vi "CRYCurve complex averaging real-time fft.vi"(7 "Initialize (F)":bool, 8 "Exponential averaging? (F=linear)":bool, 10 "Number of averages (no change)":i32, 11 "Input curve, complex":cdb[](array[numeric]) format="%.2f") -> (3 "Averaged curve":dbl[](array[numeric]) format="%.2f")   [LabVIEW 2013]
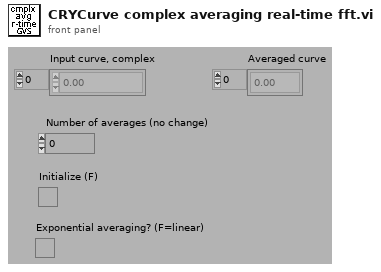
[diagram p1: front panel]
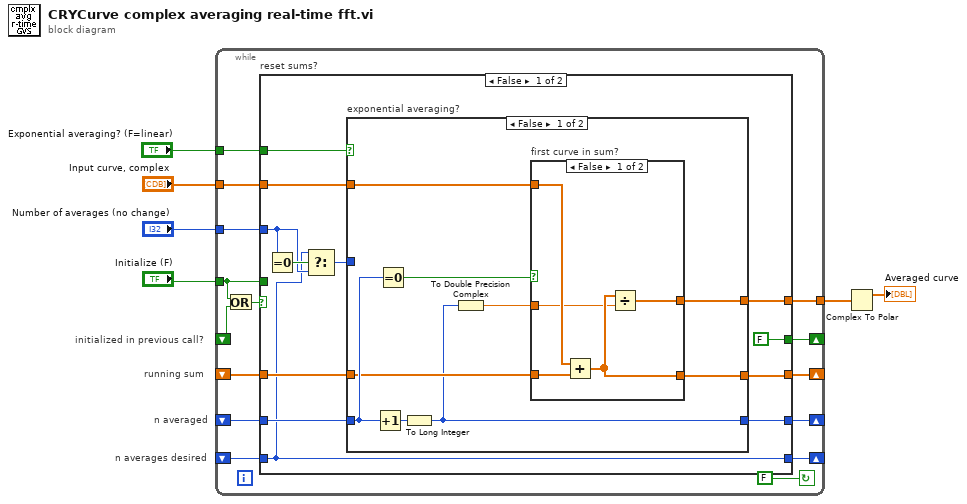
[diagram p0: block diagram]
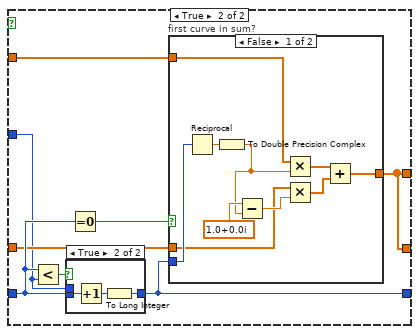
[diagram p3: hidden frame]
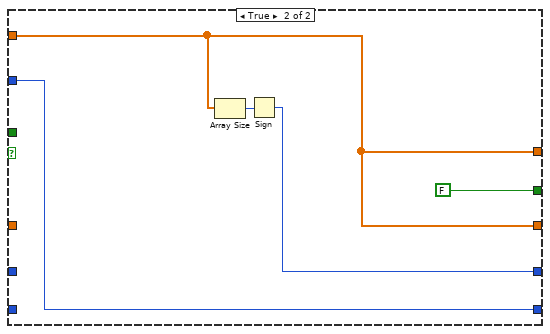
[diagram p6: hidden frame]
diagram:
  # "initialized in previous call?"
  # "n averages desired"
  # "n averaged"
  # "running sum"
  n1 = while {
    shift-left: _ -> [w9]
    shift-right: [w11] -> _
    tunnel: "Exponential averaging? (F=linear)" -> [w12]
    shift-left: _ -> [w13]
    shift-right: [w14] -> _
    tunnel: [w16] -> w2
    tunnel: "Number of averages (no change)" -> [w18]
    tunnel: "Input curve, complex" -> [w19]
    tunnel: "Initialize (F)" -> [w10]
    shift-left: _ -> [w17]
    shift-right: [w20] -> _
    shift-left: _ -> [w15]
    shift-right: [w21] -> _
    stop <- FALSE continue-if-true
    n2 = Or(x=w10, y=w9) -> (x .or. y?=w8:bool)
    n3 = case "reset sums?" shown="False" w8 {
      tunnel: [w24 w74] -> w21
      tunnel: [w30 w72] -> w20
      tunnel: w19 -> [w32 w74]
      tunnel: w18 -> [w28 w76]
      tunnel: w17 -> [w33 _]
      tunnel: [w25 w74] -> w16
      tunnel: w15 -> [w31 _]
      tunnel: [w26 w76] -> w14
      tunnel: w13 -> [w26 _]
      tunnel: w12 -> [w23 _]
      tunnel: [FALSE ("Initialize (F)") FALSE ("Initialize (F)")] -> w11
      tunnel: w10 -> [_ _]
      frame False {
        n4 = Equal To 0?(x=w28) -> (x = 0?=w29:bool)
        n5 = Select(t=w26, s=w29, f=w28) -> (s? t:f=w27:i32)
        n6 = case "exponential averaging?" shown="False" w23 {
          tunnel: w33 -> [w41 w55]
          tunnel: w32 -> [w38 w53]
          tunnel: w31 -> [w39 w52]
          tunnel: [w35 w51] -> w30
          tunnel: [w36 w49] -> w25
          tunnel: w27 -> [_ w50]
          tunnel: [w37 w49] -> w24
          frame False {
            n7 = Increment(x=w41) -> (x+1=w42:i32)
            n8 = Equal To 0?(x=w41) -> (x = 0?=w40:bool)
            n9 = To Long Integer(number=w42) -> (32bit integer=w35:i32)
            n10 = To Double Precision Complex(1:w35) -> (0:w34:cdb)
            n11 = case "first curve in sum?" shown="False" w40 {
              tunnel: w39 -> [w47 _]
              tunnel: w38 -> [w46 w48]
              tunnel: [w45 w48] -> w37
              tunnel: [w44 w48] -> w36
              tunnel: w34 -> [w43 _]
              frame False {
                n12 = Add(x=w46, y=w47) -> (x+y=w45:cdb[])
                n13 = Divide(x=w45, y=w43) -> (x/y=w44:cdb[])
              }
              frame True {
              }
            }
          }
          frame True {
            n14 = Less?(x=w55, y=w50) -> (x < y?=w56:bool)
            n15 = case shown="True" w56 {
              tunnel: w55 -> [_ w71]
              tunnel: [w68 w69] -> w51
              tunnel: w50 -> [w68 _]
              frame False {
              }
              frame True {
                n16 = Increment(x=w71) -> (x+1=w70:i32)
                n17 = To Long Integer(number=w70) -> (32bit integer=w69:i32)
              }
            }
            n18 = Equal To 0?(x=w55) -> (x = 0?=w54:bool)
            n19 = case "first curve in sum?" shown="False" w54 {
              tunnel: w53 -> [w64 w67]
              tunnel: [w59 w67] -> w49
              tunnel: w52 -> [w62 _]
              tunnel: w51 -> [w66 _]
              frame False {
                n20 = Reciprocal(x=w66) -> (1/x=w58:dbl)
                n21 = To Double Precision Complex(1:w58) -> (0:w57:cdb)
                n22 = Subtract(x=cdb 1.0+0.0i, y=w57) -> (x-y=w63:cdb)
                n23 = Multiply(x=w64, y=w57) -> (x*y=w61:cdb[])
                n24 = Multiply(x=w62, y=w63) -> (x*y=w60:cdb[])
                n25 = Add(x=w61, y=w60) -> (x+y=w59:cdb[])
              }
              frame True {
              }
            }
          }
        }
      }
      frame True {
        n26 = Array Size(array=w74) -> (size(s)=w73:i32)
        n27 = Sign(1:w73) -> (0:w72:i32)
      }
    }
  }
  n28 = Complex To Polar(r * e^(i*theta)=w2) -> (r=→"Averaged curve":dbl[])  [unwired: 1 out]
